vi "NI-Linux-RT Shared Library Path.vi"(1 "Library":T1) -> (0 "Path":path)   [LabVIEW 2020, in "common.lvlib"]
uses:
  common.lvlib
  Library Name.ctl
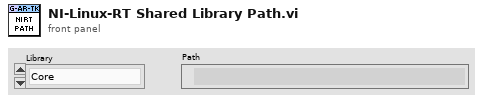
[diagram p1: front panel]
types:
  T1 = typedef "common.lvlib/Library Name.ctl" = enum16{"Core", "Feature Detection", "Augmented Reality", "DNN", "Tesseract", "Video IO"}
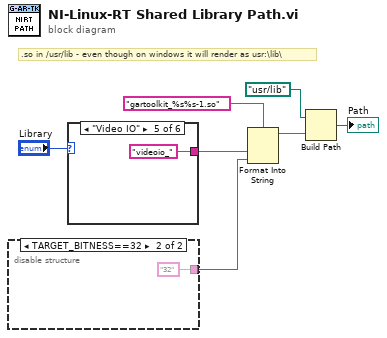
[diagram p0: block diagram]
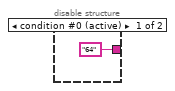
[diagram p2: hidden frame]
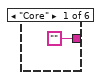
[diagram p3: hidden frame]
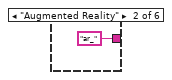
[diagram p4: hidden frame]
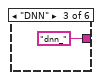
[diagram p5: hidden frame]
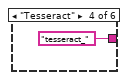
[diagram p6: hidden frame]
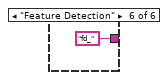
[diagram p7: hidden frame]
diagram:
  # ".so in /usr/lib - even though on windows it will render as usr:\\lib\\"
  n1 = disable-structure shown="TARGET_BITNESS==32" {
    disable-tunnel: ["64" "32"] -> w1
    frame condition #0 (active) {
    }
    frame condition #1 {
    }
  }
  n2 = case shown="\"Video IO\"" "Library" {
    tunnel: ["" "ar_" "dnn_" "tesseract_" "videoio_" "fd_"] -> w2
    frame "Core" {
    }
    frame "Augmented Reality" {
    }
    frame "DNN" {
    }
    frame "Tesseract" {
    }
    frame "Video IO" {
    }
    frame "Feature Detection" {
    }
  }
  n3 = Format Into String(format string="gartoolkit_%s%s-1.so", w2, w1) -> (resulting string=w4:string)  [unwired: 2 in, 1 out]
  n4 = Build Path(base path=path "/usr/lib", name or relative path=w4) -> (appended path=→"Path":path)
